vi "simple_udp_receiver.vi"() -> ()   [LabVIEW 2017]
uses:
  Raw Oculus Data.ctl
panel:
  out "Raw Oculus Data":T1
  in  "milliseconds to wait":u32=10
  out "error out":errorcluster
  out "String":string
  in  "stop":bool
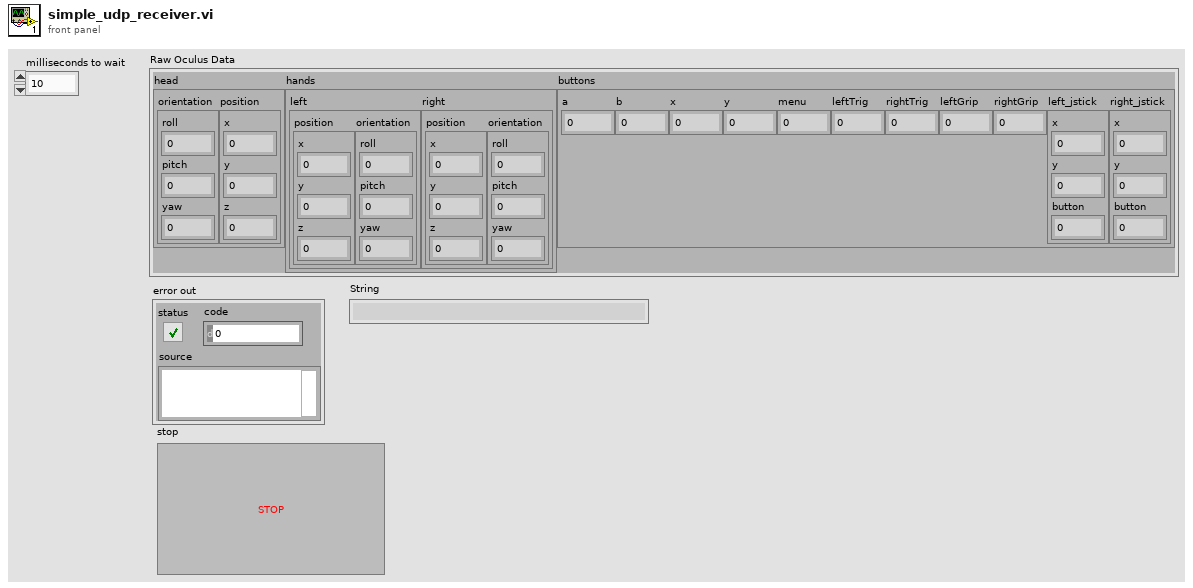
[diagram p1: front panel]
types:
  T1 = typedef "Raw Oculus Data.ctl" = cluster{"head":cluster{"orientation":cluster{"roll":dbl, "pitch":dbl, "yaw":dbl}, "position":cluster{"x":dbl, "y":dbl, "z":dbl}}, "hands":cluster{"left":cluster{"position":cluster{"x":dbl, "y":dbl, "z":dbl}, "orientation":cluster{"roll":dbl, "pitch":dbl, "yaw":dbl}}, "right":cluster{"position":cluster{"x":dbl, "y":dbl, "z":dbl}, "orientation":cluster{"roll":dbl, "pitch":dbl, "yaw":dbl}}}, "buttons":cluster{"a":i32, "b":i32, "x":i32, "y":i32, "menu":i32, "leftTrig":dbl, "rightTrig":dbl, "leftGrip":dbl, "rightGrip":dbl, "left_jstick":cluster{"x":dbl, "y":dbl, "button":i32}, "right_jstick":cluster{"x":dbl, "y":dbl, "button":i32}}}
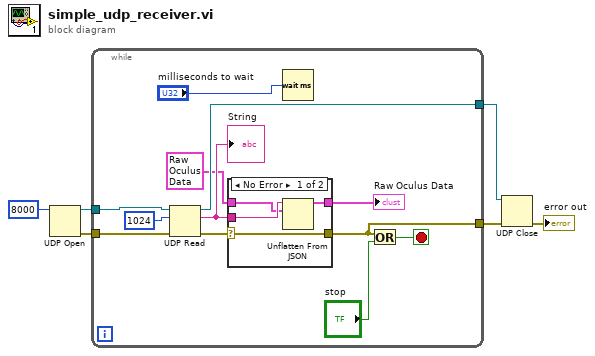
[diagram p0: block diagram]
diagram:
  n1 = UDP Open(11:8000) -> (port=w4:refnum<k16>, 0:w5:errorcluster)  [unwired: 4 in, 1 out]
  n2 = while {
    tunnel: w5 -> [w18]
    tunnel: w4 -> [w17]
    tunnel: [w16] -> w3
    tunnel: [w9] -> w1
    stop <- w14 stop-if-true
    n3 = UDP Read(connection ID=w17, max size (548)=1024, 8:w18) -> (data out=w12:string, error out=w13:errorcluster, 3:w16:refnum<k16>)  [unwired: 1 in, 2 out]
    "String" <- w12
    n4 = case shown="No Error" w13 {
      selector: w13 -> [w21 w24]
      tunnel: [w21 w24] -> w9
      tunnel: w12 -> [w22 _]
      tunnel: [w20 w23] -> w7
      tunnel: T1 {"head"={"orientation"={"roll"=0.0, "pitch"=0.0, "yaw"=0.0}, "position"={"x"=0.0, "y"=0.0, "z"=0.0}}, "hands"={"left"={"position"={"x"=0.0, "y"=0.0, "z"=0.0}, "orientation"={"roll"=0.0, "pitch"=0.0, "yaw"=0.0}}, "right"={"position"={"x"=0.0, "y"=0.0, "z"=0.0}, "orientation"={"roll"=0.0, "pitch"=0.0, "yaw"=0.0}}}, "buttons"={"a"=0, "b"=0, "x"=0, "y"=0, "menu"=0, "leftTrig"=0.0, "rightTrig"=0.0, "leftGrip"=0.0, "rightGrip"=0.0, "left_jstick"={"x"=0.0, "y"=0.0, "button"=0}, "right_jstick"={"x"=0.0, "y"=0.0, "button"=0}}} ("Raw Oculus Data") -> [w19 w23]
      frame No Error {
        n5 = Unflatten From JSON(JSON string=w22, type and defaults=w19) -> (value=w20:T1)  [unwired: 5 in, 1 out]
      }
      frame Error {
      }
    }
    "Raw Oculus Data" <- w7
    n6 = Wait (ms)(milliseconds to wait="milliseconds to wait") -> ()  [unwired: 1 out]
    n7 = Or(x=w9, y="stop") -> (x .or. y?=w14:bool)
  }
  n8 = UDP Close(connection ID=w3, 8:w1) -> (error out=→"error out":errorcluster)  [unwired: 1 out]
